vi "saveNumberedImage - Copy.vi"(8 "error in (no error)":errorcluster, 9 "Image":T1, 10 "imageNumber":u32, 11 "folder":path) -> (0 "error out":errorcluster)   [LabVIEW 2013]
uses:
  <vilib>/vision/Image Controls.llb/IMAQ Image.ctl
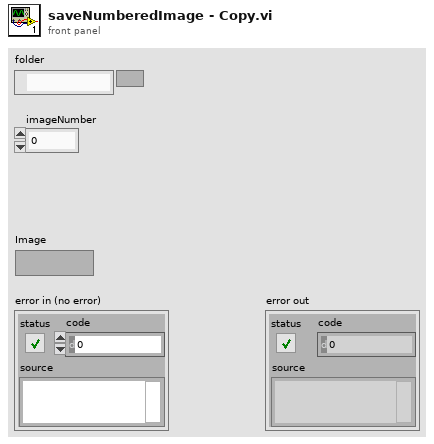
[diagram p1: front panel]
types:
  T1 = typedef "IMAQ Image.ctl" = refnum<image>
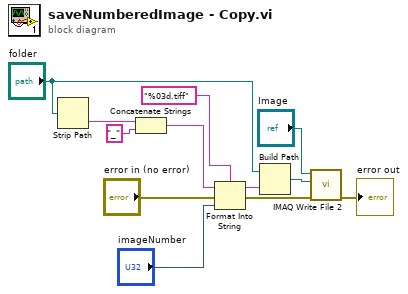
[diagram p0: block diagram]
diagram:
  n1 = Strip Path(path="folder") -> (name=w3:string)  [unwired: 1 out]
  n2 = Concatenate Strings(w3, "_" ("string")) -> (w1:string)
  n3 = Format Into String(format string="%03d.tiff", initial string=w1, error in="error in (no error)", "imageNumber") -> (resulting string=w9:string, error out=w7:errorcluster)
  n4 = Build Path(base path="folder", name or relative path=w9) -> (appended path=w8:path)
  n5 = call-poly "IMAQ Write File 2"("error in (no error)"=w7, "File Path"=w8, "Image"="Image") -> ("error out"=→"error out":errorcluster)  [unwired: 7 in, 1 out]
